vi "afmmode.vi"() -> ()   [LabVIEW 2019]
uses:
  <userlib>/Nanonis Prog Interface V5/Nanonis Prog Interface.lvlib
  <userlib>/Haptic Prog Interface/Haptic Prog Interface.lvlib
panel:
  in  "Gain":dbl=1.0 format="%_2p"
  out "force":dbl
  out "Z Write (m) 2":dbl
  in  "Z Write?":bool
  in  "Save":bool
  in  "# Sample Points":i32=4096
  out "Signal value":sgl format="%#_6p"
  out "Z Write (m)":dbl
  in  "Upper Limit (mm)":dbl=50.0
  in  "Lower Limit (mm)":dbl=-40.0
  in  "Upper Limit (nm)":dbl=1.0
  in  "Lower Limit (nm)":dbl
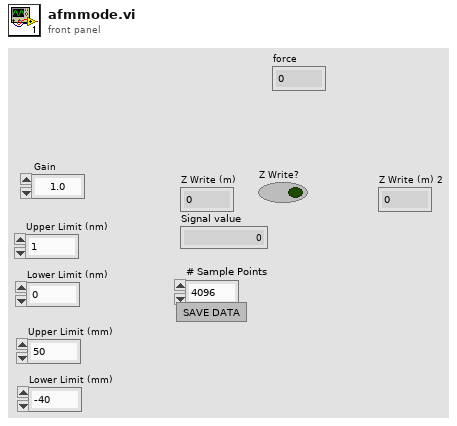
[diagram p1: front panel]
types:
  T1 = cluster{"x (mm)":dbl, "y (mm)":dbl, "z (mm)":dbl}
  T2 = cluster{"Fx (N)":dbl, "Fy (N)":dbl, "Fz (N)":dbl}
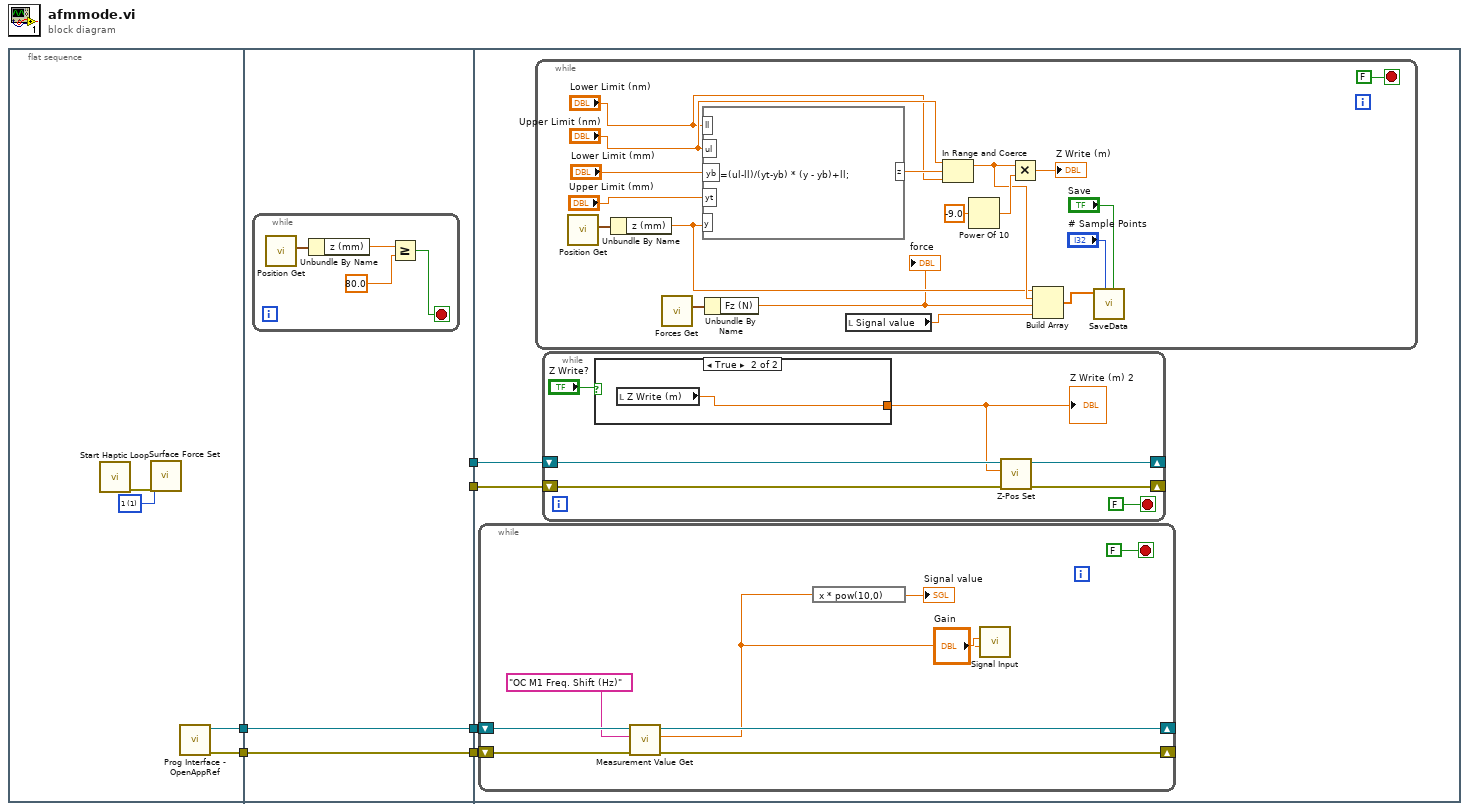
[diagram p0: block diagram]
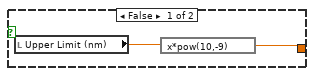
[diagram p2: hidden frame]
diagram:
  n1 = flat-sequence {
    tunnel: [w10] -> w6
    tunnel: [w9] -> w3
    tunnel: [w12] -> w5
    tunnel: [w11] -> w4
    tunnel: [w12] -> w2
    tunnel: [w11] -> w1
    tunnel: w3 -> [w11]
    tunnel: w6 -> [w12]
    tunnel: w5 -> [w20]
    tunnel: w4 -> [w19]
    tunnel: w2 -> [w18]
    tunnel: w1 -> [w17]
    frame #0 {
      w7 = u16 1 items=["0", "1", "2", "3", "4"] ("Force Settings")
      n2 = call <userlib>:"Start Haptic Loop.vi"() -> ("error out"=w8:errorcluster)  [unwired: 11 in]
      n3 = call <userlib>:"Surface Force Set.vi"("error in (no error)"=w8, "Force Settings"=w7) -> ()  [unwired: 9 in, 1 out]
      n4 = call <userlib>:"Prog Interface - OpenAppRef.vi"() -> ("Error out"=w9:errorcluster, "Application reference"=w10:refnum<vi>)  [unwired: 6 in]
    }
    frame #1 {
      n5 = while {
        stop <- w15 stop-if-true
        n6 = call <userlib>:"Position Get.vi"() -> ("Position"=w14:T1)  [unwired: 10 in, 1 out]
        n7 = Unbundle By Name(w14) -> ("z (mm)"=w13:dbl)
        n8 = Greater Or Equal?(x=w13, y=80.0) -> (x >= y?=w15:bool)
      }
    }
    frame #2 {
      n9 = while {
        shift-right: [w36] -> _
        shift-left: w20 -> [w38]
        shift-right: [w35] -> _
        shift-left: w19 -> [w37]
        stop <- FALSE stop-if-true
        n10 = call <userlib>:"Measurement Value Get.vi"("error in (no error)"=w37, "Signal Name"="OC M1 Freq. Shift (Hz)", "Application ref in"=w38) -> ("error out"=w35:errorcluster, "Measurement value"=w32:sgl, "Application ref out"=w36:refnum<vi>)  [unwired: 5 in]
        n11 = expression code="x * pow(10,0)"(w32) -> (→"Signal value":sgl)
        n12 = call <userlib>:"Signal Input.vi"("Gain"="Gain", "Signal"=w32) -> ()  [unwired: 9 in, 1 out]
      }
      n13 = while {
        stop <- FALSE stop-if-true
        n14 = call <userlib>:"Position Get.vi"() -> ("Position"=w43:T1)  [unwired: 10 in, 1 out]
        n15 = Unbundle By Name(w43) -> ("z (mm)"=w42:dbl)
        n16 = call <userlib>:"Forces Get.vi"() -> ("Force (N)"=w41:T2)  [unwired: 10 in, 1 out]
        n17 = formula code="z =(ul-ll)/(yt-yb) * (y - yb)+ll;"("ll"="Lower Limit (nm)", "ul"="Upper Limit (nm)", "yb"="Lower Limit (mm)", "yt"="Upper Limit (mm)", "y"=w42) -> ("z"=w53:dbl)
        n18 = Unbundle By Name(w41) -> ("Fz (N)"=w40:dbl)
        "force" <- w40
        n19 = local read "Signal value"() -> (w46:sgl)
        n20 = In Range and Coerce(upper limit="Upper Limit (nm)", x=w53, lower limit="Lower Limit (nm)") -> (coerced(x)=w49:dbl)  [unwired: 1 out]
        n21 = Power Of 10(x=-9.0) -> (10^x=w54:dbl)
        n22 = Multiply(x=w49, y=w54) -> (x*y=→"Z Write (m)":dbl)
        n23 = Build Array(w42, w49, w40, w46) -> (w45:dbl[])
        n24 = call "SaveData.vi"("Save"="Save", "# Sample Points"="# Sample Points", "Data"=w45) -> ()  [unwired: 9 in]
      }
      n25 = while {
        shift-right: [w23] -> _
        shift-left: w18 -> [w25]
        shift-right: [w22] -> _
        shift-left: w17 -> [w24]
        stop <- FALSE stop-if-true
        n26 = case shown="True" "Z Write?" {
          tunnel: [w28 w30] -> w21
          frame False {
            n27 = local read "Upper Limit (nm)"() -> (w29:dbl)
            n28 = expression code="x*pow(10,-9)"(w29) -> (w28:dbl)
          }
          frame True {
            n29 = local read "Z Write (m)"() -> (w30:dbl)
          }
        }
        "Z Write (m) 2" <- w21
        n30 = call <userlib>:"Z-Pos Set.vi"("error in (no error)"=w24, "Z position (m)"=w21, "Application ref in"=w25) -> ("error out"=w22:errorcluster, "Application ref out"=w23:refnum<vi>)  [unwired: 7 in]
      }
    }
  }
